vi "PH_Beckhoff_PP_Control.set i attribute.vi"(0 "i ref in":refnum<vi>, 2 "i attribute":T1={"PP Conductivity Control"={"PSDB"={"Status Service ID"=-1, "Instance ID"=-1, "Data Status"=0, "Ref Status"=refnum, "Error Code"=0}, "Status"={"GUI Ref"=refnum, "Status Service ID"=-1, "Status"=0}, "DIs"={"Device on"={"GUI Ref"=refnum, "# in Data"=-1}, "Conductivity ok"={"GUI Ref"=refnum, "# in Data"=-1}, "Temperature ok"={"GUI Ref"=refnum, "# in Data"=-1}, "Alarm"={"GUI Ref"=refnum, "# in Data"=-1}}, "PSDB Thread"={"Ref"=refnum, "Q-Ref"=refnum}}, "PP Mercury Control"={"PSDB"={"Status Service ID"=-1, "Instance ID"=-1, "Data Status"=0, "Ref Status"=refnum, "Error Code"=0}, "Status"={"GUI Ref"=refnum, "Status Service ID"=-1, "Status"=0}, "on since:"={"GUI Ref"=refnum, "Service ID"=-1, "Time"=""}, "DIs"={"Device on"={"GUI Ref"=refnum, "# in Data"=-1}, "Alarm"={"GUI Ref"=refnum, "# in Data"=-1}}, "AIs"={"Concentration"={"GUI Ref"=refnum, "# in Data"=-1}}, "PSDB Thread"={"Ref"=refnum, "Q-Ref"=refnum}}, "PSDB"={"Shot #"=-1, "Subsystem"=0}, "PSDB Credentials"={"PW"="N/A", "ID"="N/A", "DS"="N/A"}} {"PSDB"."Subsystem" items=["Miscellaneous", "fs-Frontend", "ns-Frontend", "PreAmp", "MainAmp", "MAS", "COS", "Beamline", "Experiment Laserbay", "Experiment Laserlabor", "Experiment Z6", "Timing", "Pulsed Power"]; "PP Mercury Control"."Status"."Status" items=["no info", "off/false/out", "on/true/in", "Failure", "Alarm", "Status 1", "Status 2", "Status 3"]; "PP Mercury Control"."PSDB"."Data Status" items=["no info", "no Data collection", "no problem", "Error getting the ID", "Error writing Data", "Error getting the subsystem", "Error getting the Shot ID", "Error getting the Shot Types", "Error getting the Experiments", "Error verifying wanted Shottype", "Error verifying wanted Experiment"]; "PP Conductivity Control"."Status"."Status" items=["no info", "off/false/out", "on/true/in", "Failure", "Alarm", "Status 1", "Status 2", "Status 3"]; "PP Conductivity Control"."PSDB"."Data Status" items=["no info", "no Data collection", "no problem", "Error getting the ID", "Error writing Data", "Error getting the subsystem", "Error getting the Shot ID", "Error getting the Shot Types", "Error getting the Experiments", "Error verifying wanted Shottype", "Error verifying wanted Experiment"]}, 5 "error in (no error)":errorcluster) -> (14 "i ref out":refnum<vi>, 19 "error out":errorcluster)   [LabVIEW 2014, in "PH_Beckhoff_PP_Control.lvlib"]
doc: "Sets the i attribute data of an object.\n\nLicense Agreement for this software:\n\nCopyright (C)\nGesellschaft für Schwerionenforschung, GSI\nPlanckstr. 1\n64291 Darmstadt\nGermany\n\nContact: D.Beck@gsi.de \n\nThis program is free software; you can redistribute it and/or modify it under the terms of the GNU General Public License as published by the Free Software Foundation; either version 2 of the license, or (at your option) any later version.\n\nThis program is distributed in the hope that it will be useful, but WITHOUT ANY WARRANTY; without even the implied warranty of MERCHANTABILITY or FITNESS FOR A PARTICULAR PURPOSE. See the GNU General License for more details (http://www.gnu.org).\n\nGesellschaft für Schwerionenforschung, GSI\nPlanckstr. 1, 64291 Darmstadt, Germany\nFor all questions and ideas contact: M.Richter@gsi.de, H.Brand@gsi.de or D.Beck@gsi.de.\nLast update: 17-JUN-2004"
uses:
  PH_Beckhoff_PP_Control.lvlib
  PH_Beckhoff_PP_Control.i attribute.ctl
  PH_Basics/PH_PSDBWriter/PH_PSDBWriter.Data Status.ctl
  PH_Basics/PH_StatusHandler/PH_StatusHandler.Status.ctl
  PH_Basics/PH_PSDBWriter/PH_PSDBWriter.PHELIX-Subsystems.ctl
  PH_Basics/PH_Common/Connection/PH_Connection.PSDB Credentials.ctl
  PH_Basics/PH_StatusHandler/PH_StatusHandler.lvlib
  PH_Basics/PH_PSDBWriter/PH_PSDBWriter.lvlib
  PH_Basics/PH_Common/PH_Common.lvlib
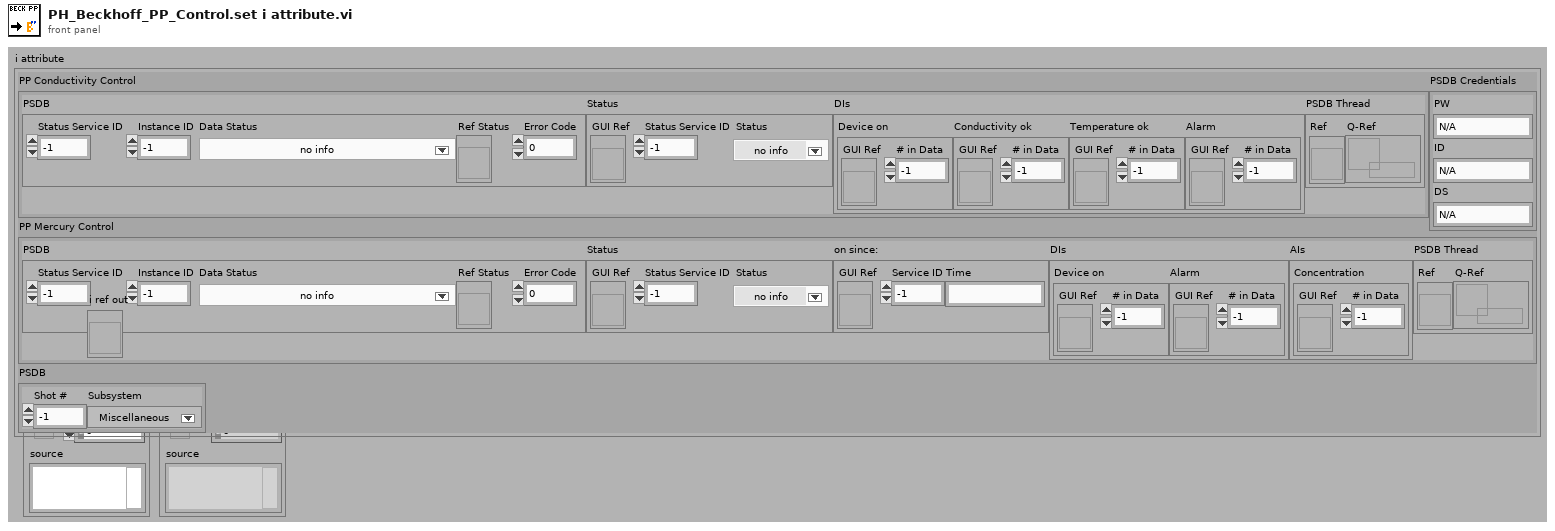
[diagram p1: front panel]
types:
  T1 = typedef "PH_Beckhoff_PP_Control.lvlib/PH_Beckhoff_PP_Control.i attribute.ctl" = cluster{"PP Conductivity Control":cluster{"PSDB":cluster{"Status Service ID":i32, "Instance ID":i32, "Data Status":T2, "Ref Status":refnum<vi>, "Error Code":i32}, "Status":cluster{"GUI Ref":refnum<vi>, "Status Service ID":i32, "Status":T3}, "DIs":cluster{"Device on":cluster{"GUI Ref":refnum<vi>, "# in Data":i32}, "Conductivity ok":cluster{"GUI Ref":refnum<vi>, "# in Data":i32}, "Temperature ok":cluster{"GUI Ref":refnum<vi>, "# in Data":i32}, "Alarm":cluster{"GUI Ref":refnum<vi>, "# in Data":i32}}, "PSDB Thread":cluster{"Ref":refnum<vi>, "Q-Ref":refnum<queue>}}, "PP Mercury Control":cluster{"PSDB":cluster{"Status Service ID":i32, "Instance ID":i32, "Data Status":T2, "Ref Status":refnum<vi>, "Error Code":i32}, "Status":cluster{"GUI Ref":refnum<vi>, "Status Service ID":i32, "Status":T3}, "on since:":cluster{"GUI Ref":refnum<vi>, "Service ID":i32, "Time":string}, "DIs":cluster{"Device on":cluster{"GUI Ref":refnum<vi>, "# in Data":i32}, "Alarm":cluster{"GUI Ref":refnum<vi>, "# in Data":i32}}, "AIs":cluster{"Concentration":cluster{"GUI Ref":refnum<vi>, "# in Data":i32}}, "PSDB Thread":cluster{"Ref":refnum<vi>, "Q-Ref":refnum<queue>}}, "PSDB":cluster{"Shot #":i32, "Subsystem":T4}, "PSDB Credentials":T5}
  T2 = typedef "PH_PSDBWriter.lvlib/PH_PSDBWriter.Data Status.ctl" = i16
  T3 = typedef "PH_StatusHandler.lvlib/PH_StatusHandler.Status.ctl" = i16
  T4 = typedef "PH_PSDBWriter.lvlib/PH_PSDBWriter.PHELIX-Subsystems.ctl" = i32
  T5 = typedef "PH_Common.lvlib/PH_Connection.PSDB Credentials.ctl" = cluster{"PW":string, "ID":string, "DS":string}
  T6 = enum16{"SetAttribute", "GetAttribute", "CreateAttribute", "DestroyAttribute", "DestroyAllAtributes"}
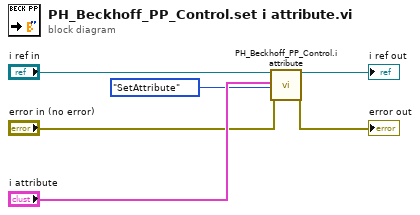
[diagram p0: block diagram]
diagram:
  n1 = call "PH_Beckhoff_PP_Control.i attribute.vi"("VI Refnum"="i ref in", "CLASS.i attribute"="i attribute", "Action"=T6."SetAttribute", "error in (no error)"="error in (no error)") -> ("VI Refnum out"=→"i ref out":refnum<vi>, "error out"=→"error out":errorcluster)  [unwired: 13 in, 1 out]
